vi "Power (1 Channel).vi"(10 "current waveform":waveform(dbl), 11 "voltage waveform":waveform(dbl)) -> (3 "power value":T1)   [LabVIEW 2017]
uses:
  <vilib>/Analysis/coordinate.llb/Angle Units.ctl
  <vilib>/Analysis/coordinate.llb/Angle Range (Degree).ctl
  <vilib>/Analysis/coordinate.llb/Wrap Angle (scalar).vi
  <vilib>/measure/matone.llb/Extract Single Tone Information 1 Chan.vi
  <vilib>/measure/NI_MAPro.lvlib
  <vilib>/Analysis/NI_AAL_Angle.lvlib
panel:
  out "Phase 2":dbl format="%.2p"
  out "Phase 1":dbl format="%.2p"
  out "detected frequency":dbl format="%.2p"
  out "Phase Diff":dbl
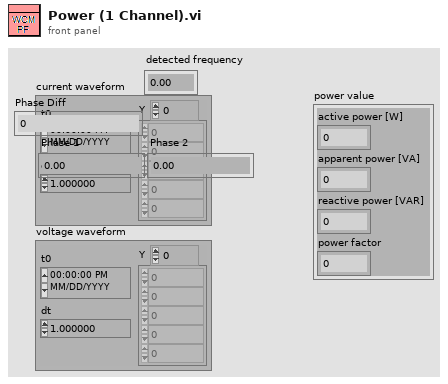
[diagram p1: front panel]
types:
  T1 = cluster{"active power [W]":dbl, "apparent power [VA]":dbl, "reactive power [VAR]":dbl, "power factor":dbl}
  T2 = typedef "NI_AAL_Angle.lvlib/Angle Range (Degree).ctl" = u16
  T3 = typedef "NI_AAL_Angle.lvlib/Angle Units.ctl" = i32
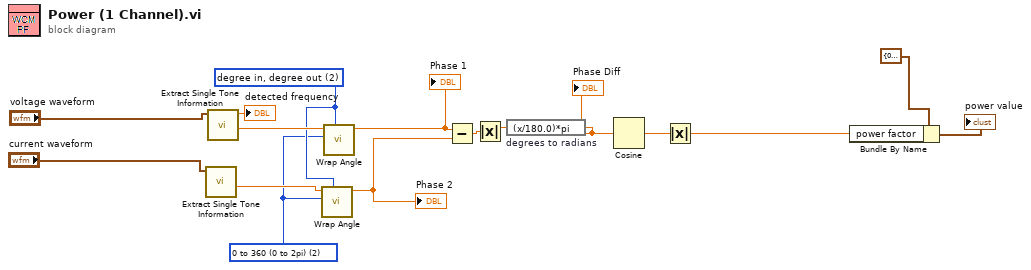
[diagram p0: block diagram]
diagram:
  w6 = T2 2 items=["none", "-180 to 180 (-pi to pi)", "0 to 360 (0 to 2pi)"] ("angle range")
  w9 = T3 2 items=["radian in, radian out", "radian in, degree out", "degree in, degree out", "degree in, radian out"] ("angle units")
  n1 = call-poly <vilib>:"Extract Single Tone Information.vi"("time signal in"="current waveform") -> ("detected phase (deg)"=w10:dbl)  [unwired: 5 in, 5 out]
  n2 = call-poly <vilib>:"Extract Single Tone Information.vi"("time signal in"="voltage waveform") -> ("detected phase (deg)"=w11:dbl, "detected frequency"=→"detected frequency":dbl)  [unwired: 5 in, 4 out]
  n3 = call-poly <vilib>:"Wrap Angle.vi"("angle units"=w9, "angle range"=w6, "angle in"=w10) -> ("angle out"=w7:dbl)  [unwired: 7 in, 1 out]
  "Phase 2" <- w7
  n4 = call-poly <vilib>:"Wrap Angle.vi"("angle units"=w9, "angle range"=w6, "angle in"=w11) -> ("angle out"=w8:dbl)  [unwired: 7 in, 1 out]
  "Phase 1" <- w8
  n5 = Subtract(x=w8, y=w7) -> (x-y=w14:dbl)
  n6 = Absolute Value(x=w14) -> (abs(x)=w5:dbl)
  n7 = expression code="(x/180.0)*pi" "degrees to radians"(w5) -> (w4:dbl)
  "Phase Diff" <- w4
  n8 = Cosine(x=w4) -> (cos(x)=w13:dbl)
  n9 = Absolute Value(x=w13) -> (abs(x)=w1:dbl)
  n10 = Bundle By Name(cluster=T1 {"active power [W]"=0.0, "apparent power [VA]"=0.0, "reactive power [VAR]"=0.0, "power factor"=0.0} ("power value"), "power factor"=w1) -> (→"power value":T1)
